vi "BeginFinish.vi"(11 "Enum":enum16{"Start", "Run", "End"}(ring)) -> ()   [LabVIEW 2012]
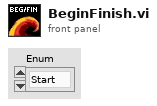
[diagram p1: front panel]
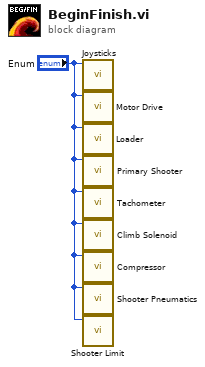
[diagram p0: block diagram]
diagram:
  n1 = call "Joysticks.vi"("Enum"="Enum") -> ()  [unwired: 9 in, 2 out]
  n2 = call "Motor Drive.vi"("Enum"="Enum") -> ()  [unwired: 11 in]
  n3 = call "Loader.vi"("Enum"="Enum") -> ()  [unwired: 10 in]
  n4 = call "Primary Shooter.vi"("Enum"="Enum") -> ()  [unwired: 11 in]
  n5 = call "Tachometer.vi"("Enum"="Enum") -> ()  [unwired: 10 in, 1 out]
  n6 = call "Climb Solenoid.vi"("Enum"="Enum") -> ()  [unwired: 11 in]
  n7 = call "Compressor.vi"("Enum"="Enum") -> ()  [unwired: 11 in]
  n8 = call "Shooter Pneumatics.vi"("Enum"="Enum") -> ()  [unwired: 10 in, 1 out]
  n9 = call "Shooter Limit.vi"("Enum"="Enum") -> ()  [unwired: 10 in, 1 out]
